vi "Rangesolver(SubVI).vi"() -> (2 "XY Graph":cluster{"X":dbl, "Y":dbl}[](graph), 3 "new picture":picture)   [LabVIEW 2024]
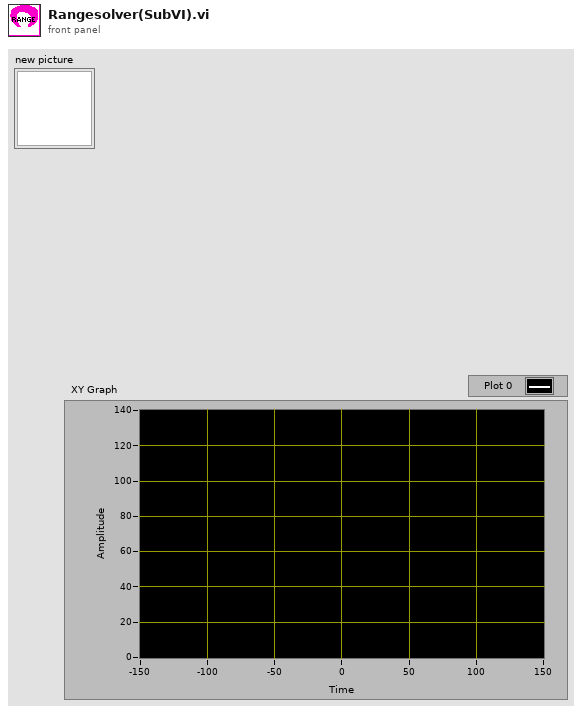
[diagram p1: front panel]
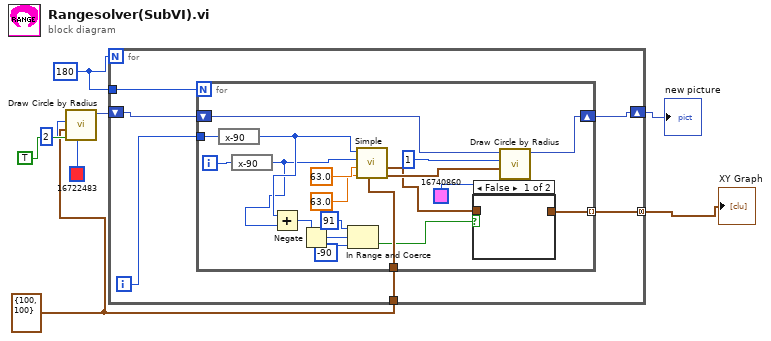
[diagram p0: block diagram]
diagram:
  w3 = cluster{"horizontal":i16, "vertical":i16} {"horizontal"=100, "vertical"=100} ("pixel center")
  w4 = 180
  n1 = call <vilib>:"Draw Circle by Radius.vi"("color(black)"=u32 16722483, "fill?(F)"=TRUE, "pixel center"=w3, "radius"=i16 2) -> ("new picture"=w5:picture)  [unwired: 7 in]
  n2 = for {
    N: w4 -> [_]
    tunnel: w4 -> [w14]
    shift-right: [w12] -> w2
    shift-left: w5 -> [w13]
    tunnel: w3 -> [w11]
    tunnel: [w9] -> w1 mode=concatenating
    i -> [w10]
    n3 = for {
      N: w14 -> [_]
      shift-right: [w26] -> w12
      shift-left: w13 -> [w27]
      tunnel: w11 -> [w28]
      tunnel: w10 -> [w25]
      tunnel: [w16] -> w9 mode=indexing
      i -> [w29]
      n4 = expression code="x-90"(w25) -> (w23:i32)
      n5 = expression code="x-90"(w29) -> (w22:i32)
      n6 = Add(x=w23, y=w22) -> (x+y=w21:i32)
      n7 = Negate(x=w21) -> (-x=w20:i32)
      n8 = In Range and Coerce(upper limit=91, x=w20, lower limit=-90) -> (In Range?=w17:bool)  [unwired: 1 out]
      n9 = call <userlib>:"Simple.vi"("2D Pict origin"=w28, "L 2"=63.0, "L 1"=63.0, "Angle 2"=w22, "Angle1"=w23) -> ("Final 2D Pos"=w24:cluster{dbl, dbl}, "end effector"=w15:cluster{dbl, dbl})  [unwired: 4 in, 1 out]
      n10 = case shown="False" w17 {
        tunnel: [_ w34] -> w16
        tunnel: w15 -> [_ w34]
        frame False {
        }
        frame True {
        }
      }
      n11 = call <vilib>:"Draw Circle by Radius.vi"("color(black)"=u32 16740860, "pixel center"=w24, "radius"=i16 1, "picture"=w27) -> ("new picture"=w26:picture)  [unwired: 7 in]
    }
  }
  "XY Graph" <- w1
  "new picture" <- w2
